vi "Get_UI_exportName.vi"(8 "error in (no error)":errorcluster, 11 "AB_Source_ExportedVI in":refnum<class "AB_Source_ExportedVI.lvclass">) -> (0 "error out":errorcluster, 2 "UI_exportName":string, 3 "AB_Source_ExportedVI out":refnum<class "AB_Source_ExportedVI.lvclass">)   [LabVIEW 2020, in "AB_Source_ExportedVI.lvclass"]
uses:
  <vilib>/AppBuilder/AB_Classes/Source/ExportedVI/AB_Source_ExportedVI.lvclass
  <vilib>/AppBuilder/AB_Classes/Source/ExportedVI/AB_Source_ExportedVI.lvclass/AB_Source_ExportedVI.ctl
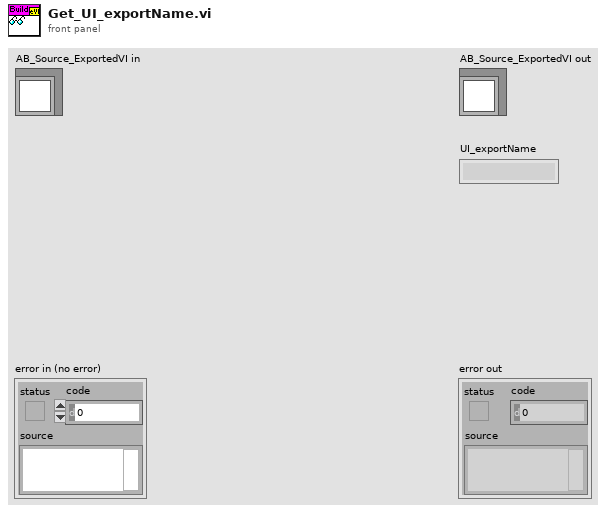
[diagram p1: front panel]
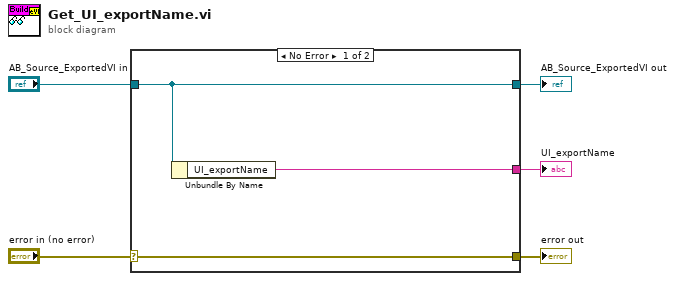
[diagram p0: block diagram]
diagram:
  n1 = case shown="No Error" "error in (no error)" {
    selector: "error in (no error)" -> [w8 w9]
    tunnel: [w8 w9] -> w4
    tunnel: [w7 w10] -> w2
    tunnel: "AB_Source_ExportedVI in" -> [w7 w10]
    tunnel: [w6 _] -> w1
    frame No Error {
      n2 = Unbundle By Name(w7) -> ("UI_exportName"=w6:string)
    }
    frame Error {
    }
  }
  "error out" <- w4
  "AB_Source_ExportedVI out" <- w2
  "UI_exportName" <- w1
